vi "Configure DUT Thermocoupler.vi"(8 "error in (no error)":errorcluster, 10 "DUT Sensor Type":T1(ring), 11 "Temperature Control in":refnum<class "Temperature Control.lvclass">) -> (0 "error out":errorcluster, 3 "Temperature Control out":refnum<class "Temperature Control.lvclass">)   [LabVIEW 2020, in "Temperature Control.lvclass"]
doc: "Configures the DUT thermocoupler"
uses:
  Temperature Control.lvclass
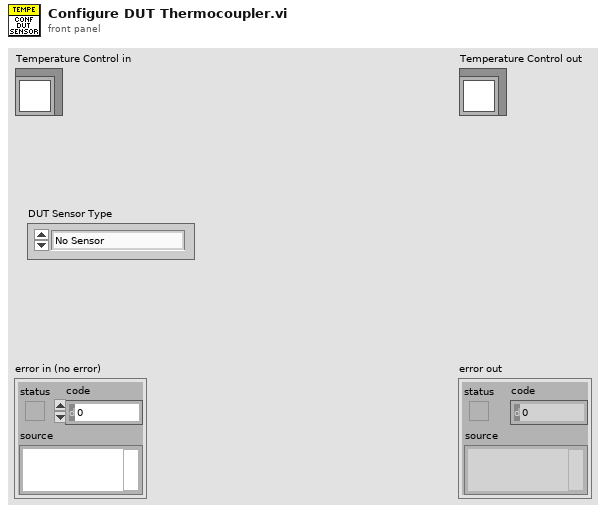
[diagram p1: front panel]
types:
  T1 = enum16{"No Sensor", "Type K Thermocoupler", "Type T Thermocoupler"}
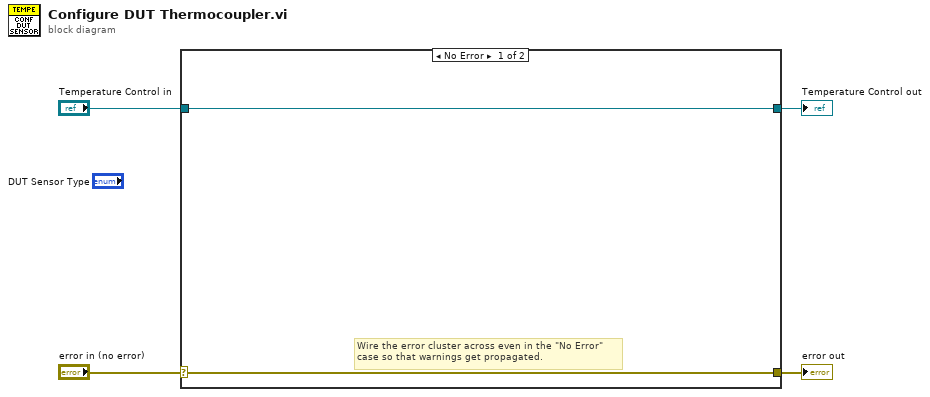
[diagram p0: block diagram]
diagram:
  n1 = case shown="No Error" "error in (no error)" {
    selector: "error in (no error)" -> [w5 w8]
    tunnel: [w5 w8] -> w3
    tunnel: [w6 w7] -> w1
    tunnel: "Temperature Control in" -> [w6 w7]
    frame No Error {
      # "Wire the error cluster across even in the \"No Error\"\ncase so that warnings get propagated."
    }
    frame Error {
    }
  }
  "error out" <- w3
  "Temperature Control out" <- w1
